vi "ExcelLabelCreation.vi"(7 "NumberOfMeasurements":i32, 8 "Error In":errorcluster, 9 "Part Name":string, 10 "AllPartInfoArray":T1=[{"PartName"="", "NumberOfRacks"=0, "MeasurementIDsArray"=[], "MeasurementNamesArray"=[], "SpecValuesArray"=[]}], 11 "TableName":string) -> (0 "Error Out":errorcluster, 3 "Labels":string[][](array[string]))   [LabVIEW 2019, in "DataLogger.lvclass"]
uses:
  DataLogger.lvclass
  Common/Controls/AllPartInfo.ctl
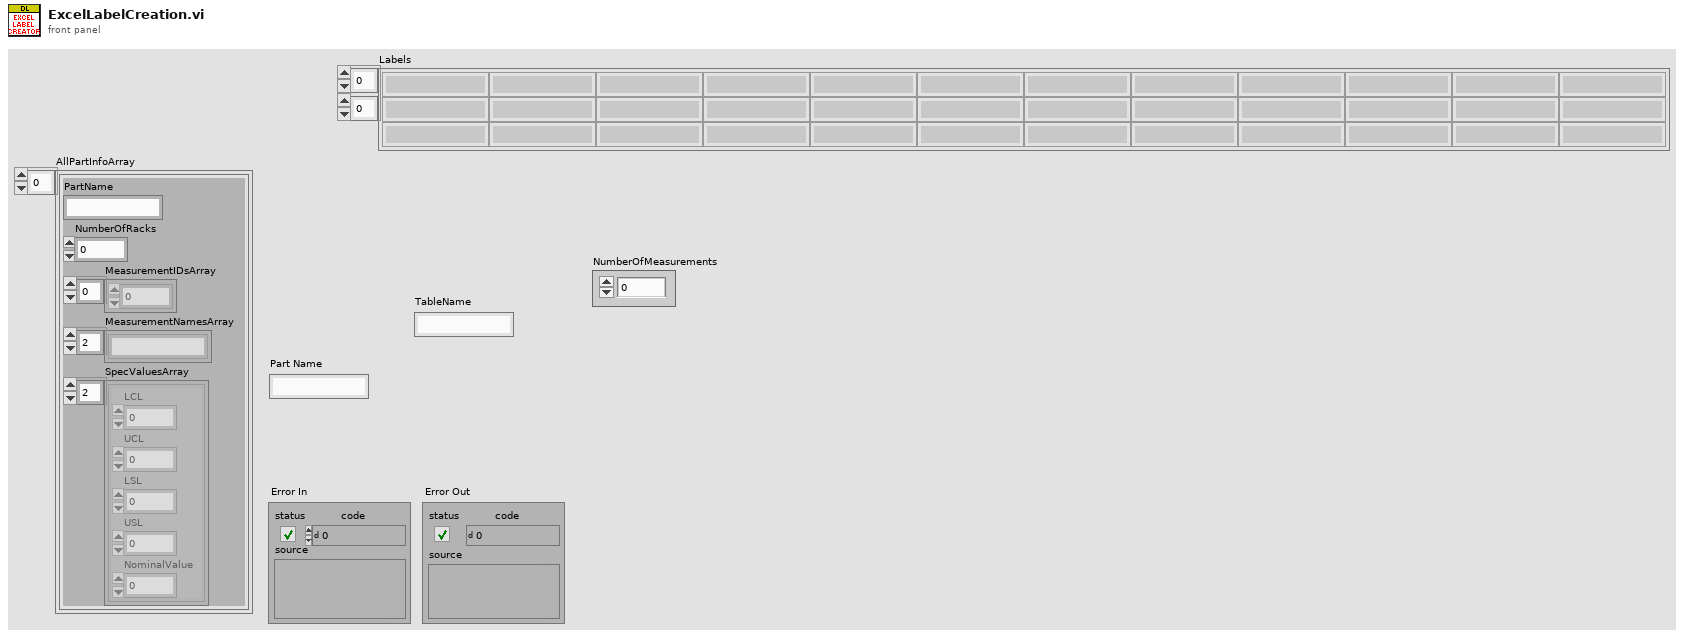
[diagram p1: front panel]
types:
  T1 = typedef "AllPartInfo.ctl" = cluster{"PartName":string, "NumberOfRacks":u8, "MeasurementIDsArray":u16[], "MeasurementNamesArray":string[], "SpecValuesArray":cluster{"LCL":dbl, "UCL":dbl, "LSL":dbl, "USL":dbl, "NominalValue":dbl}[]}[]
  T2 = cluster{"LCL":dbl, "UCL":dbl, "LSL":dbl, "USL":dbl, "NominalValue":dbl}[]
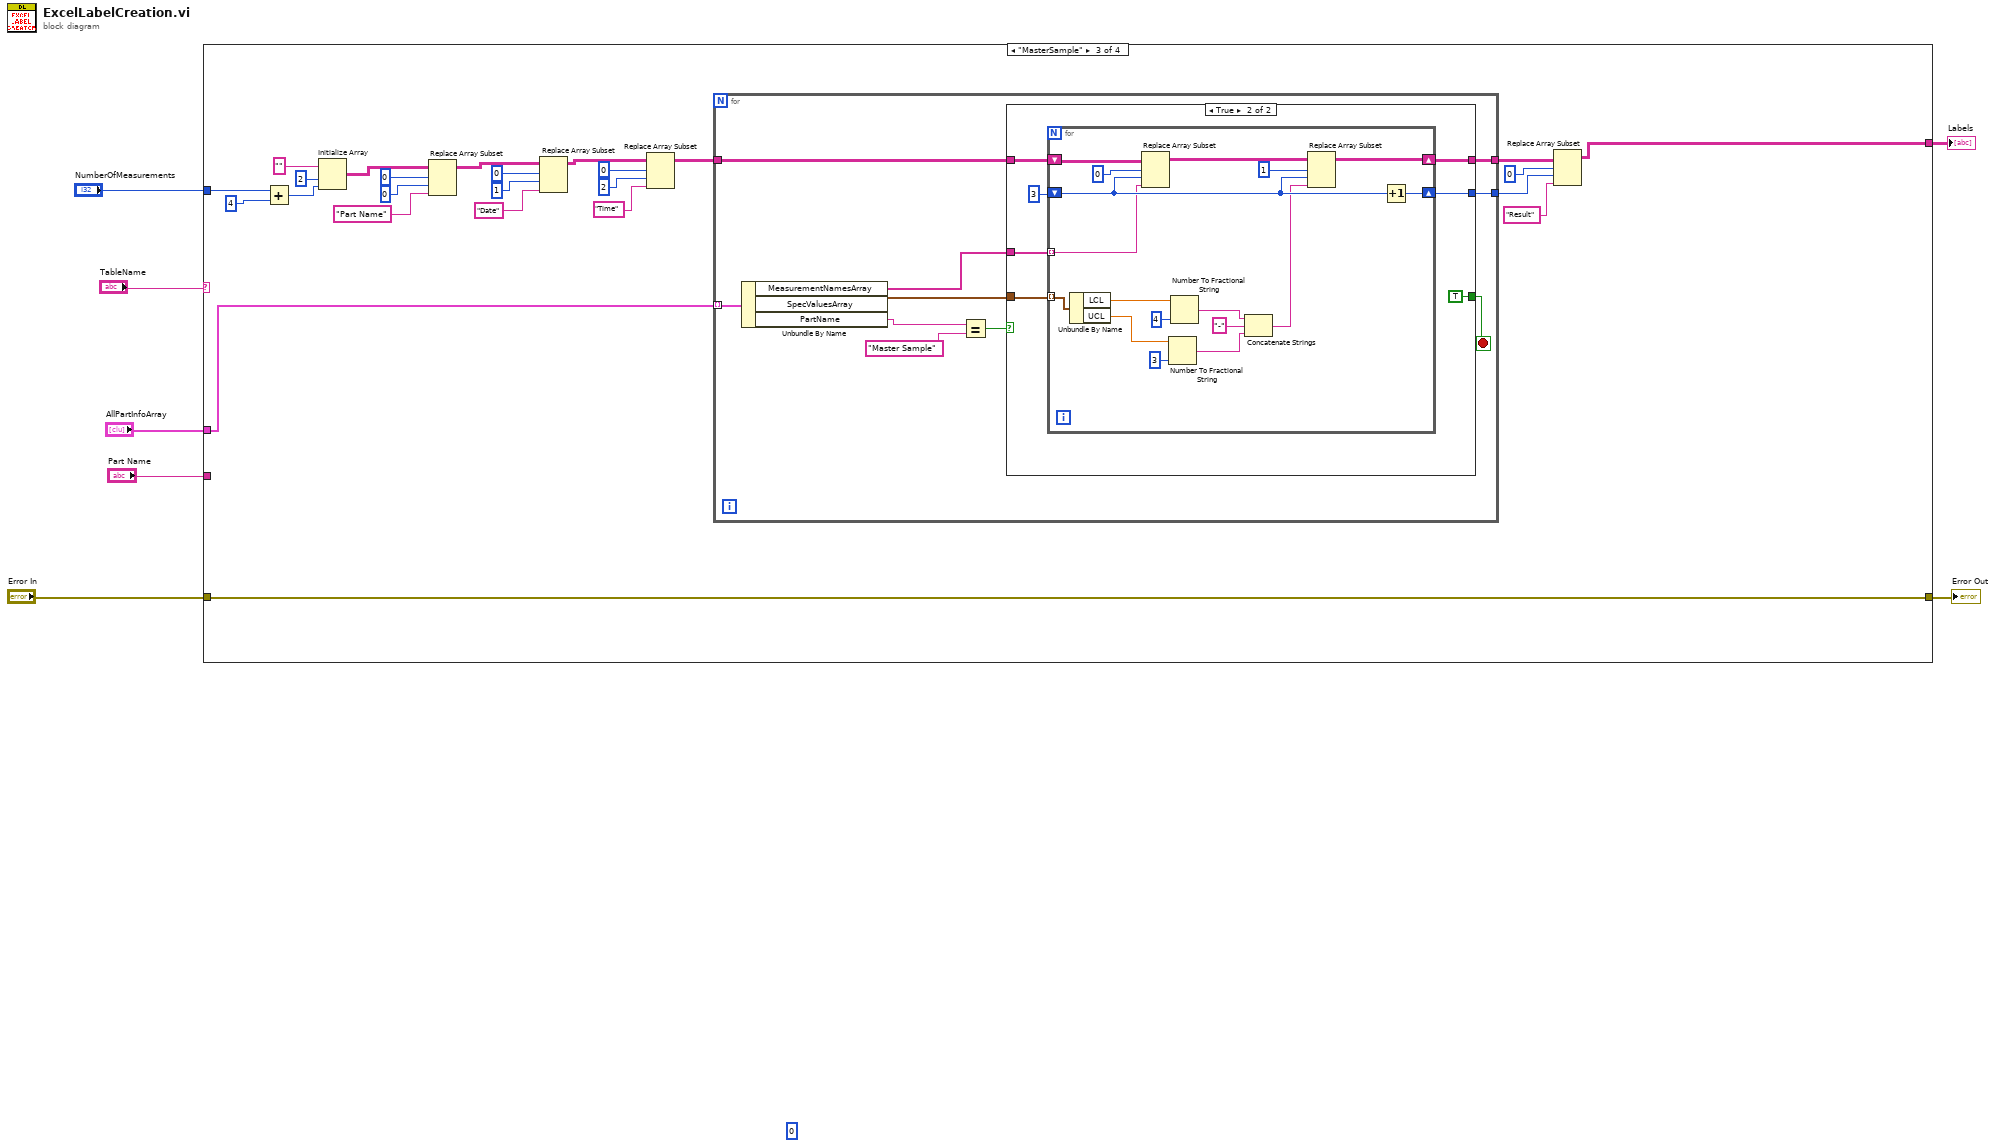
[diagram p0: block diagram]
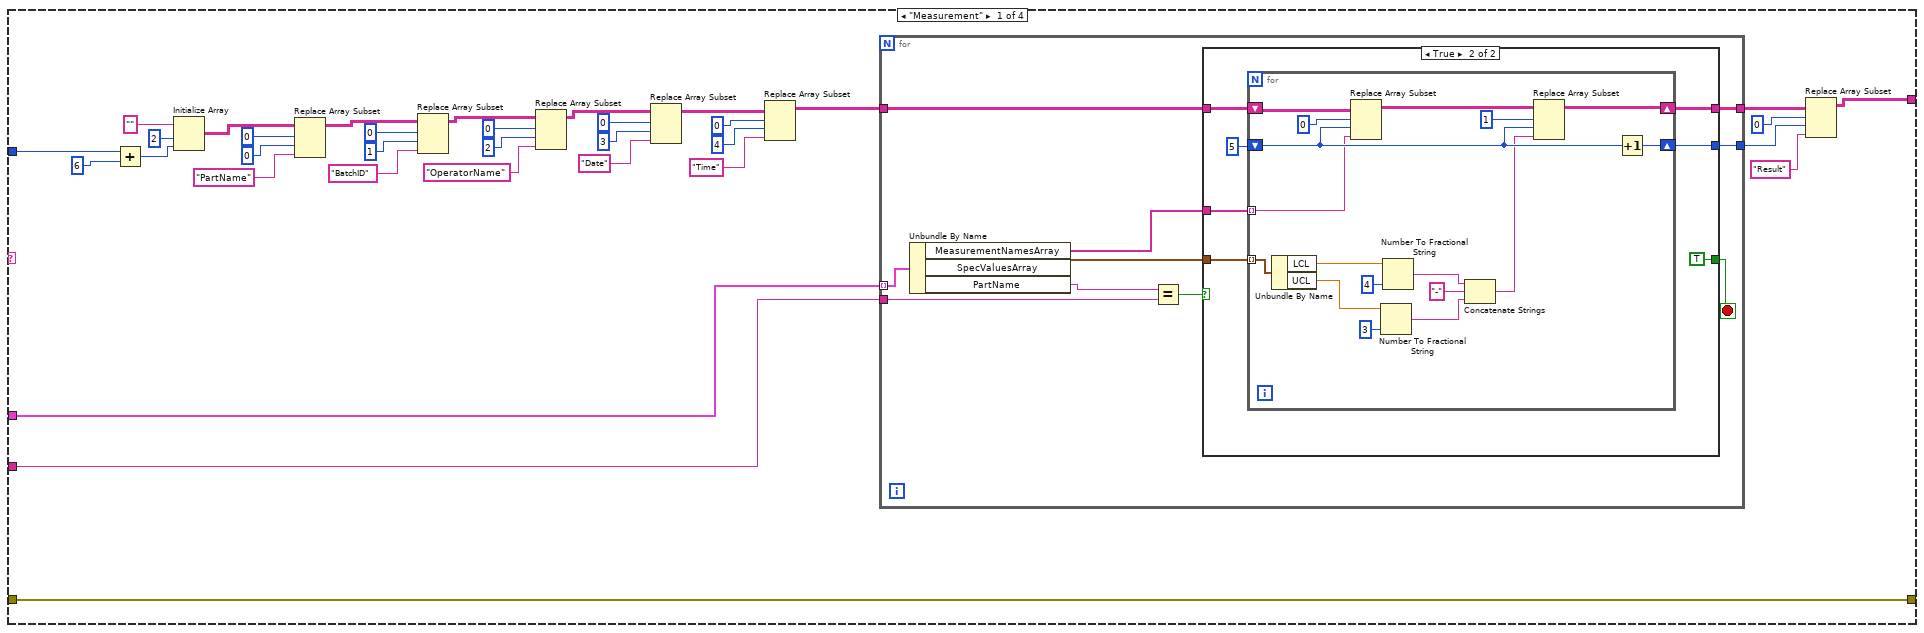
[diagram p2: hidden frame]
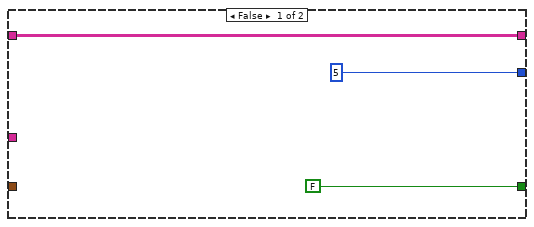
[diagram p3: hidden frame]
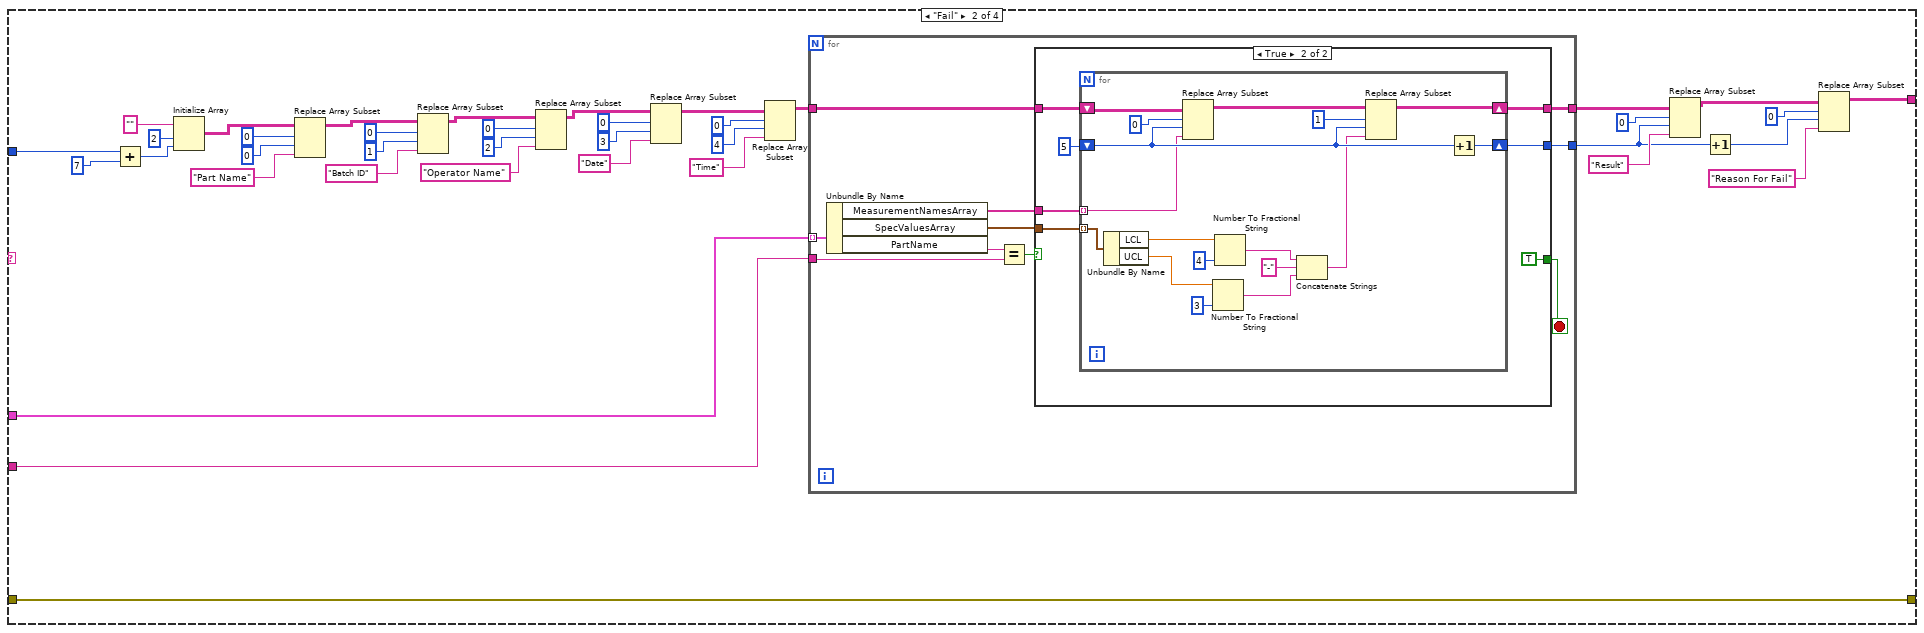
[diagram p4: hidden frame]
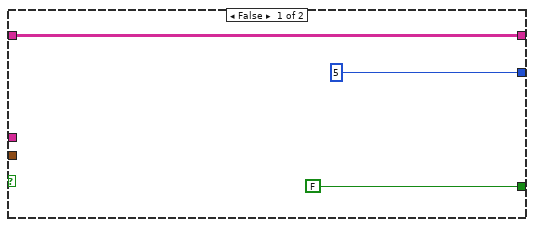
[diagram p5: hidden frame]
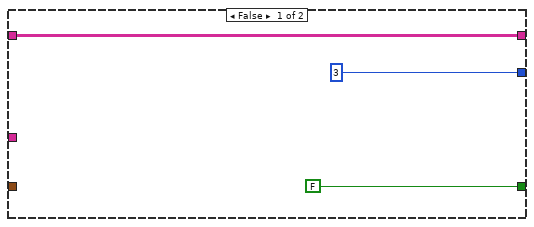
[diagram p6: hidden frame]
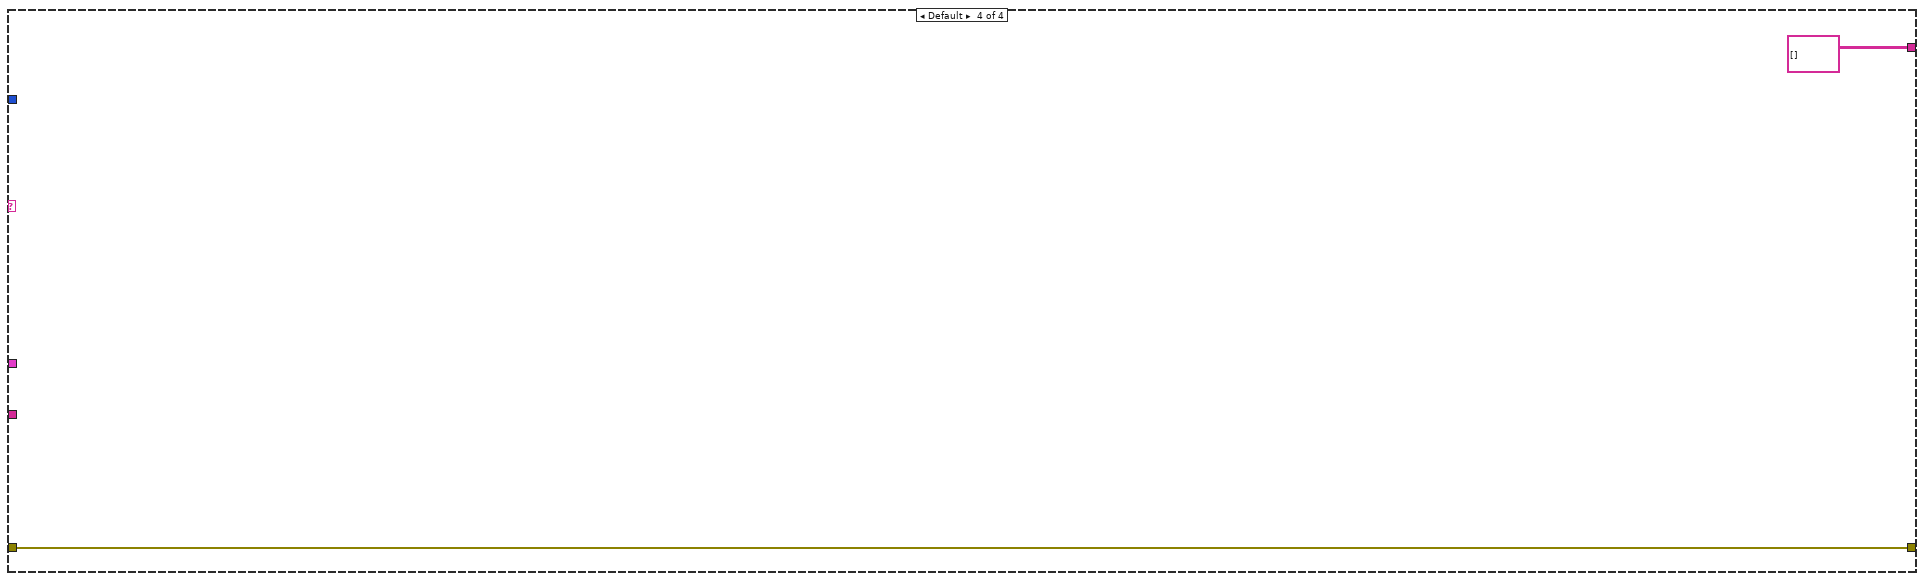
[diagram p7: hidden frame]
diagram:
  (unwired) 0
  n1 = case shown="\"MasterSample\"" "TableName" {
    tunnel: "AllPartInfoArray" -> [w15 w90 w157 _]
    tunnel: "Part Name" -> [w14 w89 _ _]
    tunnel: "NumberOfMeasurements" -> [w37 w112 w162 _]
    tunnel: [w9 w85 w154 w217] -> w2
    tunnel: "Error In" -> [w9 w85 w154 w217]
    tunnel: [w8 w79 w155 string[][] []] -> w1
    frame "Measurement" {
      n2 = Add(x=w37, y=6 ("dimension size")) -> (x+y=w39:i32)
      n3 = Initialize Array("", 2 ("dimension size"), w39) -> (w36:string[][])
      n4 = Replace Array Subset(array=w36, new element="PartName" ("new element/subarray"), index (row)=0, index (col)=0 ("disabled index (col)")) -> (w19:string[][])
      n5 = Replace Array Subset(array=w19, new element="BatchID" ("new element/subarray"), index (row)=0, index (col)=1 ("disabled index (col)")) -> (w18:string[][])
      n6 = Replace Array Subset(array=w18, new element="OperatorName" ("new element/subarray"), index (row)=0, index (col)=2 ("disabled index (col)")) -> (w17:string[][])
      n7 = Replace Array Subset(array=w17, new element="Date" ("new element/subarray"), index (row)=0, index (col)=3 ("disabled index (col)")) -> (w20:string[][])
      n8 = Replace Array Subset(array=w20, new element="Time" ("new element/subarray"), index (row)=0, index (col)=4 ("disabled index (col)")) -> (w16:string[][])
      n9 = for {
        tunnel: w16 -> [w51]
        tunnel: w15 -> [w44] mode=indexing
        tunnel: w14 -> [w47]
        tunnel: [w46] -> w11
        tunnel: [w45] -> w10
        stop <- w50 stop-if-true
        n10 = Unbundle By Name(w44) -> ("MeasurementNamesArray"=w42:string[], "SpecValuesArray"=w43:T2, "PartName"=w48:string)
        n11 = Equal?(x=w48, y=w47) -> (x = y?=w49:bool)
        n12 = case shown="True" w49 {
          tunnel: w51 -> [w53 w61]
          tunnel: [FALSE TRUE] -> w50
          tunnel: [w53 w58] -> w46
          tunnel: [5 ("disabled index (col)") w57] -> w45
          tunnel: w43 -> [_ w56]
          tunnel: w42 -> [_ w55]
          frame False {
          }
          frame True {
            n13 = for {
              shift-right: [w63] -> w58
              shift-left: w61 -> [w77]
              shift-right: [w76] -> w57
              shift-left: 5 ("disabled index (col)") -> [w68]
              tunnel: w56 -> [w75] mode=indexing
              tunnel: w55 -> [w62] mode=indexing
              n14 = Unbundle By Name(w75) -> ("LCL"=w74:dbl, "UCL"=w73:dbl)
              n15 = Replace Array Subset(array=w77, new element=w62, index (row)=0, index (col)=w68) -> (w69:string[][])
              n16 = Number To Fractional String(number=w73, precision (6)=i16 3) -> (F-format string=w65:string)  [unwired: 2 in]
              n17 = Number To Fractional String(number=w74, precision (6)=i16 4) -> (F-format string=w67:string)  [unwired: 2 in]
              n18 = Concatenate Strings(w67, "-" ("string"), w65) -> (w64:string)
              n19 = Replace Array Subset(array=w69, new element=w64, index (row)=1, index (col)=w68) -> (w63:string[][])
              n20 = Increment(x=w68) -> (x+1=w76:i32)
            }
          }
        }
      }
      n21 = Replace Array Subset(array=w11, new element="Result" ("new element/subarray"), index (row)=0, index (col)=w10) -> (w8:string[][])
    }
    frame "Fail" {
      n22 = Add(x=w112, y=7 ("dimension size")) -> (x+y=w114:i32)
      n23 = Initialize Array("", 2 ("dimension size"), w114) -> (w111:string[][])
      n24 = Replace Array Subset(array=w111, new element="Part Name" ("new element/subarray"), index (row)=0, index (col)=0 ("disabled index (col)")) -> (w94:string[][])
      n25 = Replace Array Subset(array=w94, new element="Batch ID" ("new element/subarray"), index (row)=0, index (col)=1 ("disabled index (col)")) -> (w93:string[][])
      n26 = Replace Array Subset(array=w93, new element="Operator Name" ("new element/subarray"), index (row)=0, index (col)=2 ("disabled index (col)")) -> (w92:string[][])
      n27 = Replace Array Subset(array=w92, new element="Date" ("new element/subarray"), index (row)=0, index (col)=3 ("disabled index (col)")) -> (w95:string[][])
      n28 = Replace Array Subset(array=w95, new element="Time" ("new element/subarray"), index (row)=0, index (col)=4 ("disabled index (col)")) -> (w91:string[][])
      n29 = for {
        tunnel: w91 -> [w126]
        tunnel: w90 -> [w119] mode=indexing
        tunnel: w89 -> [w122]
        tunnel: [w121] -> w86
        tunnel: [w120] -> w81
        stop <- w125 stop-if-true
        n30 = Unbundle By Name(w119) -> ("MeasurementNamesArray"=w117:string[], "SpecValuesArray"=w118:T2, "PartName"=w123:string)
        n31 = Equal?(x=w123, y=w122) -> (x = y?=w124:bool)
        n32 = case shown="True" w124 {
          tunnel: w126 -> [w128 w136]
          tunnel: [FALSE TRUE] -> w125
          tunnel: [w128 w133] -> w121
          tunnel: [5 ("disabled index (col)") w132] -> w120
          tunnel: w118 -> [_ w131]
          tunnel: w117 -> [_ w130]
          frame False {
          }
          frame True {
            n33 = for {
              shift-right: [w138] -> w133
              shift-left: w136 -> [w152]
              shift-right: [w151] -> w132
              shift-left: 5 ("disabled index (col)") -> [w143]
              tunnel: w131 -> [w150] mode=indexing
              tunnel: w130 -> [w137] mode=indexing
              n34 = Unbundle By Name(w150) -> ("LCL"=w149:dbl, "UCL"=w148:dbl)
              n35 = Replace Array Subset(array=w152, new element=w137, index (row)=0, index (col)=w143) -> (w144:string[][])
              n36 = Number To Fractional String(number=w148, precision (6)=i16 3) -> (F-format string=w140:string)  [unwired: 2 in]
              n37 = Number To Fractional String(number=w149, precision (6)=i16 4) -> (F-format string=w142:string)  [unwired: 2 in]
              n38 = Concatenate Strings(w142, "-" ("string"), w140) -> (w139:string)
              n39 = Replace Array Subset(array=w144, new element=w139, index (row)=1, index (col)=w143) -> (w138:string[][])
              n40 = Increment(x=w143) -> (x+1=w151:i32)
            }
          }
        }
      }
      n41 = Replace Array Subset(array=w86, new element="Result" ("new element/subarray"), index (row)=0, index (col)=w81) -> (w82:string[][])
      n42 = Increment(x=w81) -> (x+1=w80:i32)
      n43 = Replace Array Subset(array=w82, new element="Reason For Fail" ("new element/subarray"), index (row)=0, index (col)=w80) -> (w79:string[][])
    }
    frame "MasterSample" {
      n44 = Add(x=w162, y=4 ("dimension size")) -> (x+y=w176:i32)
      n45 = Initialize Array("", 2 ("dimension size"), w176) -> (w174:string[][])
      n46 = Replace Array Subset(array=w174, new element="Part Name" ("new element/subarray"), index (row)=0, index (col)=0 ("disabled index (col)")) -> (w164:string[][])
      n47 = Replace Array Subset(array=w164, new element="Date" ("new element/subarray"), index (row)=0, index (col)=1 ("disabled index (col)")) -> (w163:string[][])
      n48 = Replace Array Subset(array=w163, new element="Time" ("new element/subarray"), index (row)=0, index (col)=2 ("disabled index (col)")) -> (w156:string[][])
      n49 = for {
        tunnel: w156 -> [w188]
        tunnel: w157 -> [w182] mode=indexing
        tunnel: [w184] -> w159
        tunnel: [w183] -> w158
        stop <- w187 stop-if-true
        n50 = Unbundle By Name(w182) -> ("MeasurementNamesArray"=w180:string[], "SpecValuesArray"=w181:T2, "PartName"=w185:string)
        n51 = Equal?(x=w185, y="Master Sample") -> (x = y?=w186:bool)
        n52 = case shown="True" w186 {
          tunnel: w188 -> [w190 w198]
          tunnel: [FALSE TRUE] -> w187
          tunnel: [w190 w195] -> w184
          tunnel: [3 ("disabled index (col)") w194] -> w183
          tunnel: w181 -> [_ w193]
          tunnel: w180 -> [_ w192]
          frame False {
          }
          frame True {
            n53 = for {
              shift-right: [w200] -> w195
              shift-left: w198 -> [w214]
              shift-right: [w213] -> w194
              shift-left: 3 ("disabled index (col)") -> [w205]
              tunnel: w193 -> [w212] mode=indexing
              tunnel: w192 -> [w199] mode=indexing
              n54 = Unbundle By Name(w212) -> ("LCL"=w211:dbl, "UCL"=w210:dbl)
              n55 = Replace Array Subset(array=w214, new element=w199, index (row)=0, index (col)=w205) -> (w206:string[][])
              n56 = Number To Fractional String(number=w210, precision (6)=i16 3) -> (F-format string=w202:string)  [unwired: 2 in]
              n57 = Number To Fractional String(number=w211, precision (6)=i16 4) -> (F-format string=w204:string)  [unwired: 2 in]
              n58 = Concatenate Strings(w204, "-" ("string"), w202) -> (w201:string)
              n59 = Replace Array Subset(array=w206, new element=w201, index (row)=1, index (col)=w205) -> (w200:string[][])
              n60 = Increment(x=w205) -> (x+1=w213:i32)
            }
          }
        }
      }
      n61 = Replace Array Subset(array=w159, new element="Result" ("new element/subarray"), index (row)=0, index (col)=w158) -> (w155:string[][])
    }
    frame Default {
    }
  }
  "Error Out" <- w2
  "Labels" <- w1
